vi "GetInstrument type.vi"(0 "object in":refnum<class "WK6440B.lvclass">, 5 "error in (no error)":errorcluster) -> (14 "object out":refnum<class "WK6440B.lvclass">, 15 "Instrument type":enum16{""}(ring), 19 "error out":errorcluster)   [LabVIEW 2013, in "WK6440B.lvclass"]
uses:
  WK6440B.lvclass
  WK6440B.lvclass/WK6440B.ctl
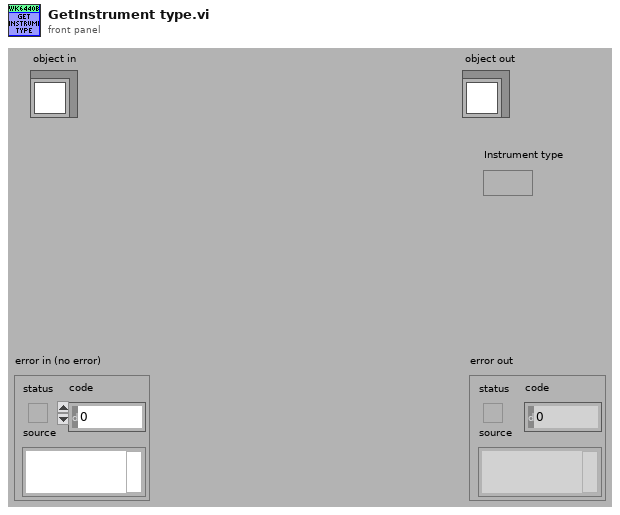
[diagram p1: front panel]
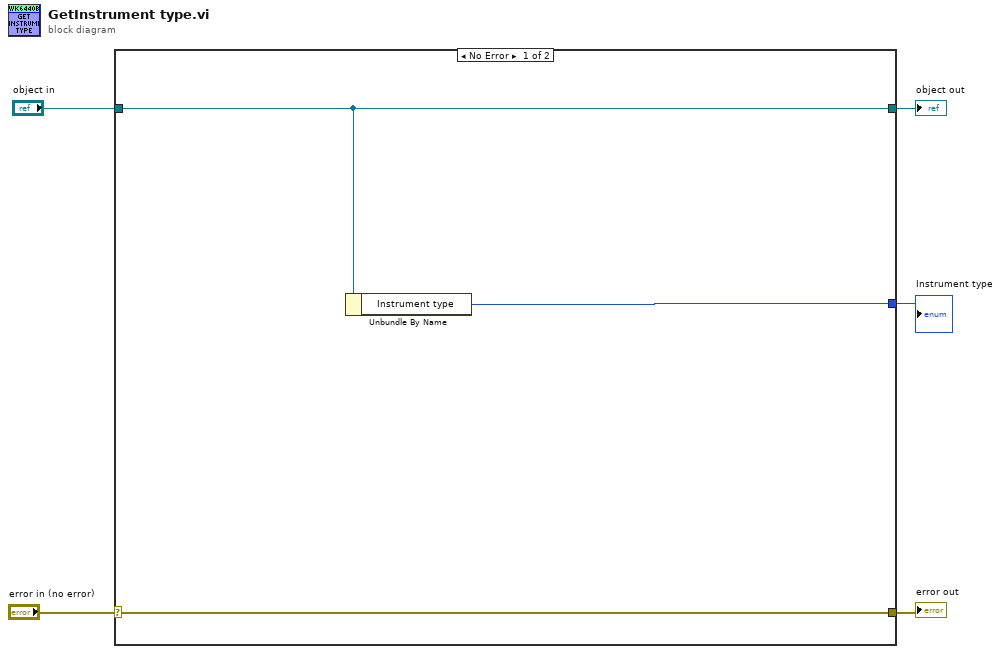
[diagram p0: block diagram]
diagram:
  n1 = case shown="No Error" "error in (no error)" {
    selector: "error in (no error)" -> [w7 w10]
    tunnel: [w7 w10] -> w4
    tunnel: [w6 w9] -> w2
    tunnel: "object in" -> [w6 w9]
    tunnel: [w8 _] -> w1
    frame No Error {
      n2 = Unbundle By Name(w6) -> ("Instrument type"=w8:enum16{""})
    }
    frame Error {
    }
  }
  "error out" <- w4
  "object out" <- w2
  "Instrument type" <- w1
